vi "FIRE_SUPPRESSION_SAFETY_INTERLOCK.vi"(3 "Fire":bool) -> (0 "CO2 Flooding in Progress":bool, 1 "Fire Detector-2":bool, 2 "Fire Detector-1":bool)   [LabVIEW 2014]
panel:
  # "FIRE SUPPRESSION SAFETY INTERLOCK"
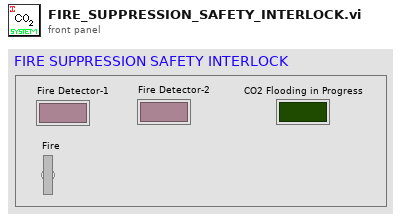
[diagram p1: front panel]
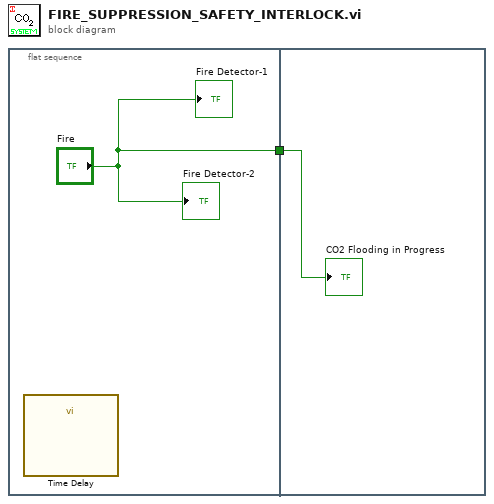
[diagram p0: block diagram]
diagram:
  n1 = flat-sequence {
    tunnel: ["Fire"] -> w1
    tunnel: w1 -> [w3]
    frame #0 {
      n2 = call "Time Delay"() -> ()  [unwired: 11 in, 1 out]
      "Fire Detector-1" <- "Fire"
      "Fire Detector-2" <- "Fire"
    }
    frame #1 {
      "CO2 Flooding in Progress" <- w3
    }
  }
